vi "m1m3_getNextSample_AccelerometerData.vi"(8 "error in (no error)":errorcluster, 11 "AccelerometerData_Ctl":T1={"Timestamp"=0.0, "RawAccelerometerX[2]"=[0.0, 0.0], "RawAccelerometerY[2]"=[0.0, 0.0], "RawAccelerometerZ[4]"=[0.0, 0.0, 0.0, 0.0], "AngularAccelerationX"=0.0, "AngularAccelerationY"=0.0, "AngularAccelerationZ"=0.0}) -> (0 "error out":errorcluster, 2 "function return":i32, 3 "AccelerometerData_Ctl out":T1)   [LabVIEW 2016, in "SALLV_m1m3.lvlib"]
doc: "int m1m3_shm_getNextSample_AccelerometerDataLV(m1m3_AccelerometerDataLV *AccelerometerData_Ctl );"
uses:
  SALLV_m1m3.lvlib
  DataTypes/AccelerometerData.ctl
  SALLV_m1m3.so
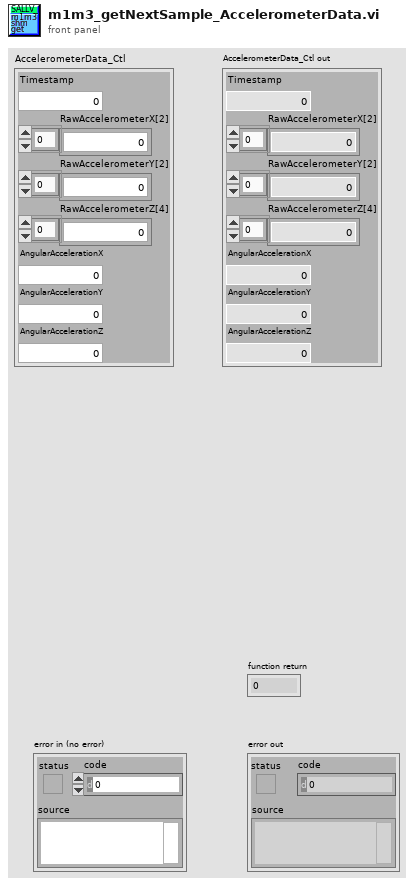
[diagram p1: front panel]
types:
  T1 = typedef "SALLV_m1m3.lvlib/AccelerometerData.ctl" = cluster{"Timestamp":dbl, "RawAccelerometerX[2]":dbl[], "RawAccelerometerY[2]":dbl[], "RawAccelerometerZ[4]":dbl[], "AngularAccelerationX":dbl, "AngularAccelerationY":dbl, "AngularAccelerationZ":dbl}
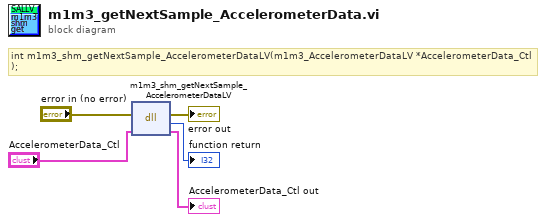
[diagram p0: block diagram]
diagram:
  # "int m1m3_shm_getNextSample_AccelerometerDataLV(m1m3_AccelerometerDataLV *AccelerometerData_Ctl );"
  n1 = dll-call lib="opt/CODE/SALLV_m1m3/SALLV_m1m3.*" fn="m1m3_shm_getNextSample_AccelerometerDataLV"(error in="error in (no error)", "AccelerometerData_Ctl"="AccelerometerData_Ctl") -> (error out=→"error out":errorcluster, →"function return":i32, "AccelerometerData_Ctl"=→"AccelerometerData_Ctl out":T1)  [unwired: 2 in, 1 out]
